vi "Balance-update.vi"(8 "error in (no error)":errorcluster, 10 "Balance":string, 11 "ATM-Controller in":refnum<class "ATM-Controller.lvclass">) -> (0 "error out":errorcluster, 3 "ATM-Controller out":refnum<class "ATM-Controller.lvclass">)   [LabVIEW 2025, in "ATM-Controller.lvlib" / "ATM-Controller.lvclass"]
uses:
  ATM-Controller.lvclass
  ATM-Controller.lvclass/ATM-Controller.ctl
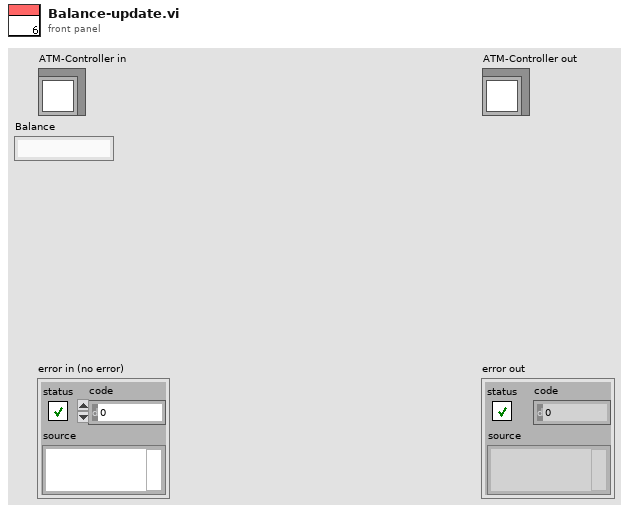
[diagram p1: front panel]
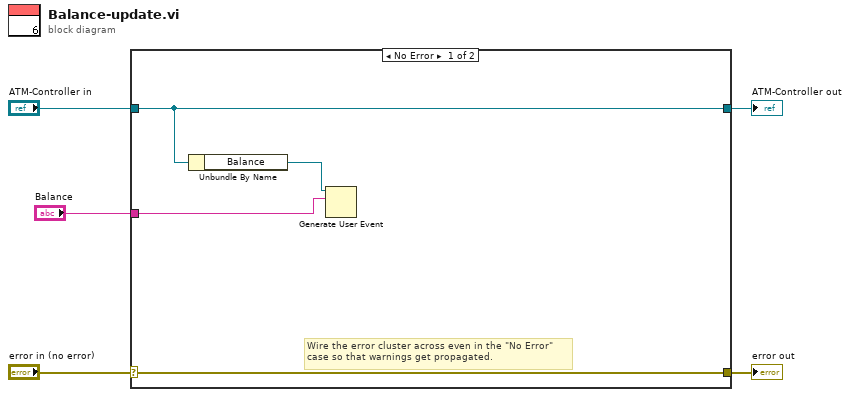
[diagram p0: block diagram]
diagram:
  n1 = case shown="No Error" "error in (no error)" {
    selector: "error in (no error)" -> [w9 w11]
    tunnel: [w9 w11] -> w4
    tunnel: [w7 w10] -> w2
    tunnel: "ATM-Controller in" -> [w7 w10]
    tunnel: "Balance" -> [w8 _]
    frame No Error {
      # "Wire the error cluster across even in the \"No Error\"\ncase so that warnings get propagated."
      n2 = Unbundle By Name(w7) -> ("Balance"=w6:refnum<user-event>)
      n3 = Generate User Event(user event=w6, event data cluster=w8) -> ()  [unwired: 2 in, 2 out]
    }
    frame Error {
    }
  }
  "error out" <- w4
  "ATM-Controller out" <- w2
